vi "Generate Pitch Waveform_1P.vi"(8 "Error In":errorcluster, 11 "Pitch Frequency":dbl=2200.0 format="%#_13g") -> (0 "Error Out":errorcluster, 3 "Pitch Waveform":dbl[](array[numeric]))   [LabVIEW 2014]
uses:
  <vilib>/measure/NI_MABase.lvlib
panel:
  out "Waveform Graph":dbl[](graph)
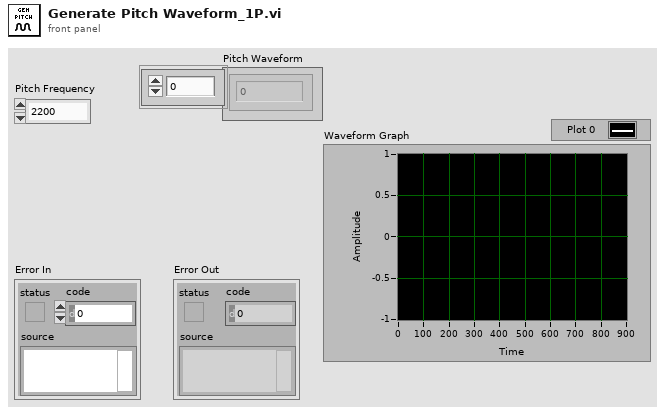
[diagram p1: front panel]
types:
  T1 = cluster{"Sampling Rate":dbl, "Number of Samples":dbl}
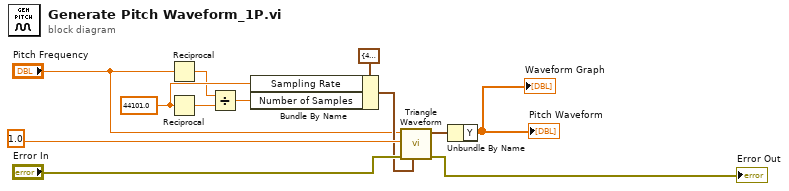
[diagram p0: block diagram]
diagram:
  w5 = 44101.0 ("x")
  n1 = Reciprocal(x="Pitch Frequency") -> (1/x=w2:dbl)
  n2 = Reciprocal(x=w5) -> (1/x=w3:dbl)
  n3 = Divide(x=w2, y=w3) -> (x/y=w7:dbl)
  n4 = Bundle By Name(cluster=T1 {"Sampling Rate"=44101.0, "Number of Samples"=201.0} ("Sampling Info"), "Sampling Rate"=w5, "Number of Samples"=w7) -> (w6:T1)
  n5 = call <vilib>:"Triangle Waveform.vi"("sampling info"=w6, "error in (no error)"="Error In", "amplitude"=1.0, "frequency"="Pitch Frequency") -> ("error out"=→"Error Out":errorcluster, "signal out"=w11:waveform(dbl))  [unwired: 6 in]
  n6 = Unbundle By Name(w11) -> ("Y"=→"Waveform Graph" →"Pitch Waveform":dbl[])
